vi "Format Message New to Old.vi"(7 "Raw Message In":string) -> (8 "Conv Message Out":string)   [LabVIEW 2023, in "GEA2_Toolkit.lvlib"]
uses:
  library/GEA2_Toolkit.lvlib
  <vilib>/Utility/error.llb/Trim Whitespace One-Sided.vi
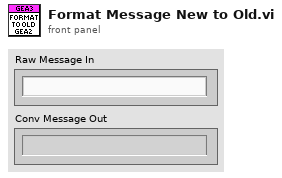
[diagram p1: front panel]
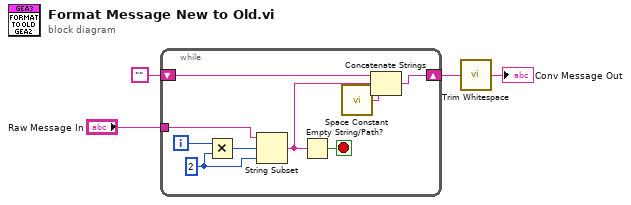
[diagram p0: block diagram]
diagram:
  n1 = while {
    shift-right: [w11] -> w1
    shift-left: "" -> [w12]
    tunnel: "Raw Message In" -> [w7]
    i -> [w10]
    stop <- w5 stop-if-true
    w8 = 2 ("y")
    n2 = Multiply(x=w10, y=w8) -> (x*y=w9:i32)
    n3 = String Subset(string=w7, offset (0)=w9, length (rest)=w8) -> (substring=w6:string)
    n4 = Empty String/Path?(string/path=w6) -> (empty?=w5:bool)
    n5 = call <vilib>:"Space Constant.vi"() -> ("String"=w13:string)
    n6 = Concatenate Strings(w12, w6, w13) -> (w11:string)
  }
  n7 = call <vilib>:"Trim Whitespace.vi"("string"=w1) -> ("trimmed string"=→"Conv Message Out":string)  [unwired: 1 in]
